vi "AMC Feedback Message.vi"(4 "timeout in ms (5000)":i32=5000, 6 "Reply":variant, 7 "Result":variant, 8 "error in (no error)":errorcluster, 9 "Messages":string, 10 "Reply Data Type":T1, 11 "Model_AMC in":refnum<class "Model_AMC.lvclass">) -> (0 "error out":errorcluster, 3 "Model_AMC out":refnum<class "Model_AMC.lvclass">)   [LabVIEW 2021, in "Model_AMC.lvclass"]
uses:
  Model_AMC.lvclass
  <userlib>/John_Lib/AMC_FW/AMC_SelfCustom/Reply Data Type.ctl
  <userlib>/John_Lib/AMC_FW/AMC_SelfCustom/Message Type.ctl
  Model_AMC.lvclass/Model_AMC.ctl
  <userlib>/John_Lib/AMC_FW/AMC_FW.lvlib
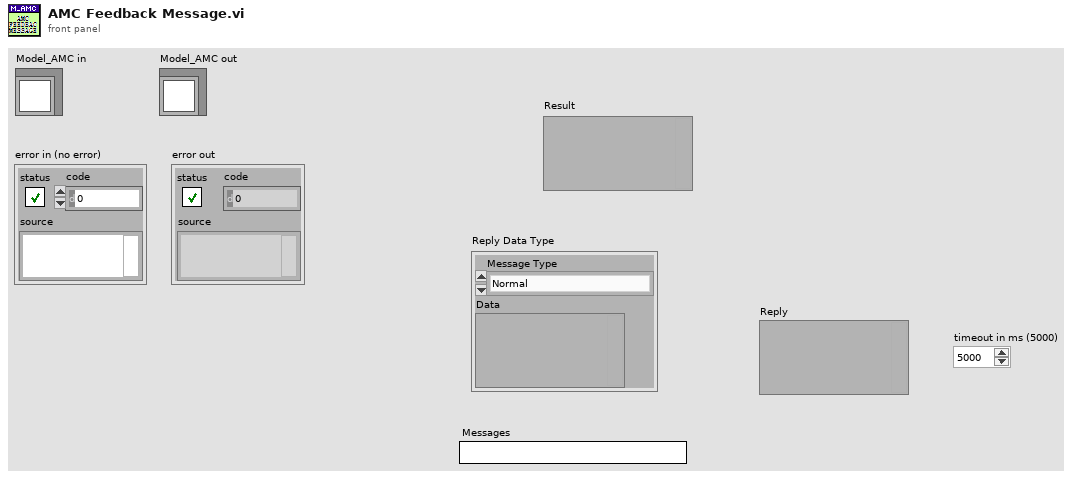
[diagram p1: front panel]
types:
  T1 = typedef "AMC_FW.lvlib/Reply Data Type.ctl" = cluster{"Message Type":T2, "Data":variant}
  T2 = typedef "AMC_FW.lvlib/Message Type.ctl" = enum16{"Normal", "AMC_Reply", "OPCUA", "NetworkSteam"}
  T3 = typedef "Model_AMC.lvclass/DVR.ctl" = cluster{"JKI_Network_Streams":refnum<class "NetworkConnection.lvclass">, "AMC Q":T4, "Connnected":bool}
  T4 = typedef "Model_AMC.lvclass/AMC Q.ctl" = cluster{"Main":T5, "OPCUA":T5, "NetworkSteam":T5}
  T5 = typedef "AMC_FW.lvlib/Queue.ctl" = cluster{"Q":T6, "Name":string}
  T6 = typedef "AMC_FW.lvlib/Message Queue.ctl" = refnum<queue>
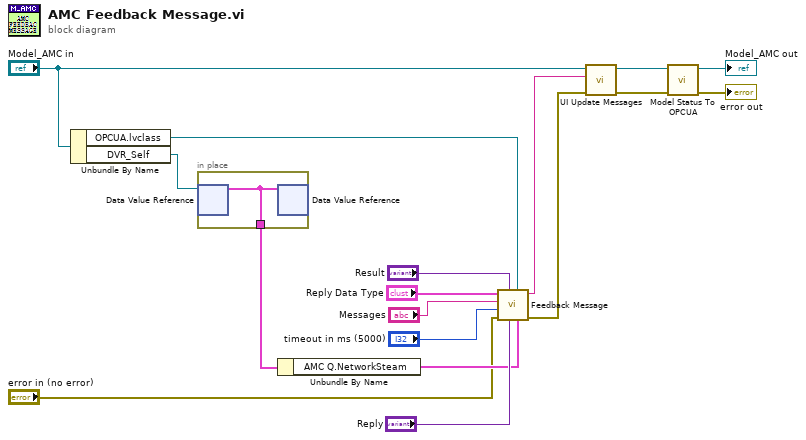
[diagram p0: block diagram]
diagram:
  n1 = Unbundle By Name("Model_AMC in") -> ("OPCUA.lvclass"=w9:refnum<class "OPCUA.lvclass">, "DVR_Self"=w16:refnum<data-value>)
  n2 = in-place {
    in-place-border: [w18] -> w17
    n3 = in-place-dvr #1(w16) -> (w18:T3)  [unwired: 1 out]
    n4 = in-place-dvr #1(w18) -> ()  [unwired: 2 out]
  }
  n5 = Unbundle By Name(w17) -> ("AMC Q.NetworkSteam"=w10:T5)
  n6 = call <userlib>:"Feedback Message.vi"("AMC Q.NetworkSteam"=w10, "OPCUA.lvclass"=w9, "Reply"="Reply", "Result"="Result", "error in (no error)"="error in (no error)", "timeout in ms (5000)"="timeout in ms (5000)", "Messages"="Messages", "Reply Data Type"="Reply Data Type") -> ("error out"=w2:errorcluster, "Messages Out"=w6:string)  [unwired: 2 in]
  n7 = call "UI Update Messages.vi"("error in (no error)"=w2, "UserMessage"=w6, "Model_AMC in"="Model_AMC in") -> ("error out"=w1:errorcluster, "Model_AMC out"=w4:refnum<class "Model_AMC.lvclass">)  [unwired: 7 in]
  n8 = call "Model Status To OPCUA.vi"("error in (no error)"=w1, "Model_AMC in"=w4) -> ("error out"=→"error out":errorcluster, "Model_AMC out"=→"Model_AMC out":refnum<class "Model_AMC.lvclass">)  [unwired: 8 in]
